vi "Zone.vi"(7 "error source vi name":string, 8 "error in (no error)":errorcluster, 11 "Pointer in":refnum<class "Pointer.lvclass">) -> (0 "error out":errorcluster, 3 "Pointer out":refnum<class "Pointer.lvclass">)   [LabVIEW 2016, in "Memory Manager.lvlib" / "Pointer.lvclass"]
uses:
  Pointer.lvclass
  Errors.ctl
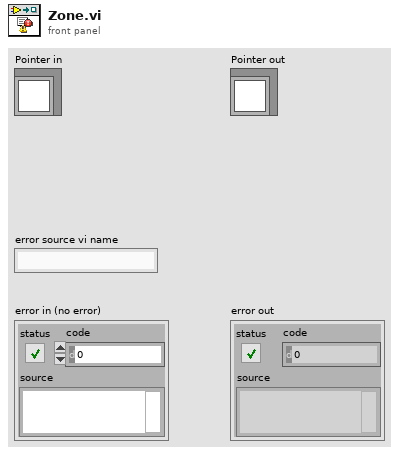
[diagram p1: front panel]
types:
  T1 = typedef "Memory Manager.lvlib/Pointer.lvclass/Errors.ctl" = enum16{"No Error", "Null Pointer", "Out of Bounds", "Buffer Underflow", "Size Mismatch", "Zone"}
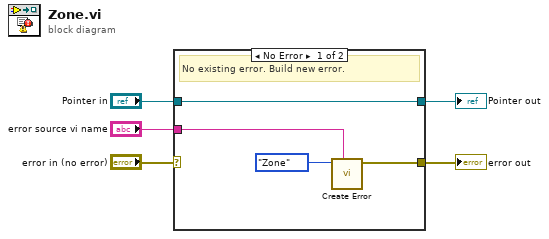
[diagram p0: block diagram]
diagram:
  n1 = case shown="No Error" "error in (no error)" {
    selector: "error in (no error)" -> [_ w11]
    tunnel: [w6 w11] -> w3
    tunnel: "error source vi name" -> [w8 _]
    tunnel: "Pointer in" -> [w7 w10]
    tunnel: [w7 w10] -> w1
    frame No Error {
      # "No existing error. Build new error."
      n2 = call "Create Error.vi"("source vi name"=w8, "error"=Errors."Zone") -> ("error out"=w6:errorcluster)  [unwired: 8 in, 1 out]
    }
    frame Error {
      # "Incoming error. Pass through."
    }
  }
  "error out" <- w3
  "Pointer out" <- w1
